vi "Handle Error.vi"(8 "error in (no error)":errorcluster, 11 "Analyze Actor in":refnum<class "Analyze Actor.lvclass">) -> (0 "error out":errorcluster, 2 "stop actor?":bool=TRUE, 3 "Analyze Actor out":refnum<class "Analyze Actor.lvclass">)   [LabVIEW 2014, in "Analyze Actor.lvlib" / "Analyze Actor.lvclass"]
doc: "(<B>Filename</B>: Actor Framework.lvlib:Actor.lvclass:Handle Error.vi)\n\nDefines how the actor handles an error that occurred while processing a message. By default, this method does nothing except stop the actor."
uses:
  Analyze Actor.lvclass
  <vilib>/ActorFramework/Actor/Actor.lvclass
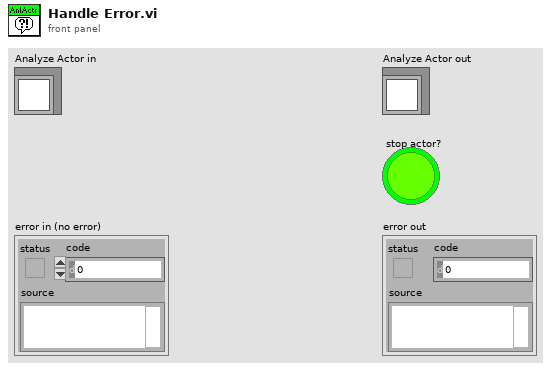
[diagram p1: front panel]
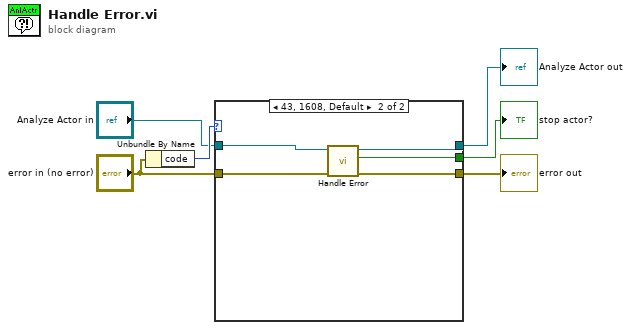
[diagram p0: block diagram]
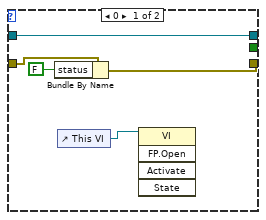
[diagram p2: hidden frame]
diagram:
  n1 = Unbundle By Name("error in (no error)") -> ("code"=w6:i32)
  n2 = case shown="43, 1608, Default" w6 {
    tunnel: [w10 w16] -> w2
    tunnel: [_ w15] -> w3
    tunnel: [w8 w14] -> w4
    tunnel: "error in (no error)" -> [w11 w13]
    tunnel: "Analyze Actor in" -> [w8 w12]
    frame 0 {
      n3 = Bundle By Name(cluster=w11, "status"=FALSE) -> (w10:errorcluster)
      n4 = control-ref of="This VI"() -> (w7:refnum<vi>)
      n5 = invoke class="VI" method="FP.Open"(reference=w7) -> ()  [unwired: 4 in, 5 out]
    }
    frame 43, 1608, Default {
      n6 = call-parent "Handle Error.vi"("error in (no error)"=w13, "Actor in"=w12) -> ("error out"=w16:errorcluster, "stop actor?"=w15:bool, "Actor out"=w14:refnum<class "Analyze Actor.lvclass">)  [unwired: 7 in]
    }
  }
  "Analyze Actor out" <- w4
  "error out" <- w2
  "stop actor?" <- w3
